vi "Panel Get Dryer Weight.vi"(0 "VISA resource name":refnum<visa-resource-name>, 2 "Agilent Scale?":bool, 11 "error in (no error)":errorcluster) -> (4 "VISA resource name out":refnum<visa-resource-name>, 6 "Empty Dryer Cold Weight":dbl, 8 "Init Scale Temp":dbl, 15 "error out":errorcluster)   [LabVIEW 2009]
uses:
  Global Test Variables DPT.vi
panel:
  out "Error Message":string
  in  "stop":bool
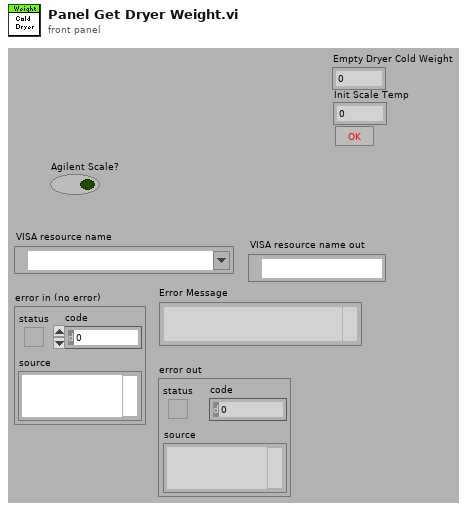
[diagram p1: front panel]
types:
  T1 = typedef "DPT Global Type.ctl" = cluster{"Test Setup":cluster{"RH Resistor":dbl, "Temp Cal":dbl, "Temp Coeff":dbl, "Power On Threshold":dbl, "MA Filter Size":i32, "Weight Offset":dbl, "Temp Resistor":dbl, "Gas Enabled":bool, "Gas P. Resistor":dbl, "Scale Com":dbl, "W. Samps":i32, "Temp4mA Val":dbl, "Temp20mA Val":dbl, "RH4mA Val":dbl, "RH20mA Val":dbl, "GPres4mA Val":dbl, "Gpres20mA Val":dbl}, "Agilent Setup":cluster{"Scale Channel":string, "TC Channels":string, "VDC Discrete Channels":string, "RH Chan":string, "Temp Chan":string, "Tscale Channel":string, "RDB Channel":string, "Gas Temperature":string, "Gas Pressure":string, "Barometric Pressure":string, "Gas Feedback Chan":string}, "Directories":cluster{"Work File Directory":path, "Save File Directory":path, "Library Directory":path, "Data Backup Directory":path, "Data Backup Dir Fail":path, "Lab Directory":path}, "Test Information":cluster{"Model:":string, "Temperature:":string, "Engineer:":string, "Technician:":string, "Comments:":string, "Lab ID:":string, "TR Number:":string, "Test Number:":string, "Test Station:":string, "Empty Dryer Cold Weight:":dbl, "Serial Number:":string, "Build:":string, "Dryer Type":string, "Humidity":string, "Test Title per TR:":string}, "cDAQ Array Locations":cluster{"Scale Channel":string, "TC Channels":string, "VDC Discrete Channel":string, "RH Chan":string, "Temp Chan":string, "Tscale Channel":string, "RDB Channel":string, "Gas Temperature":string, "Gas Pressure":string, "Barometric Pressure":string, "Gas Feedback Chan":string}}
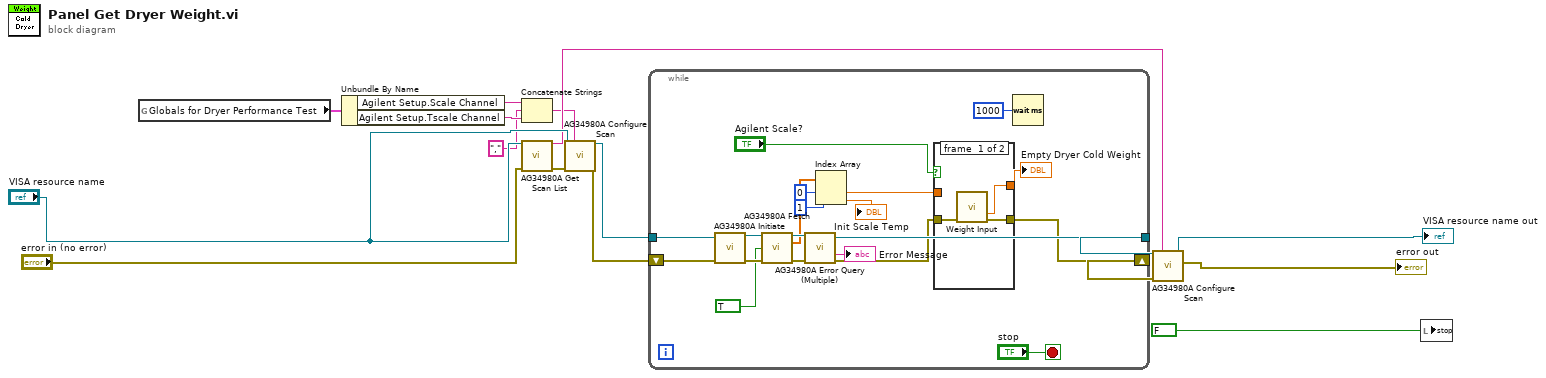
[diagram p0: block diagram]
diagram:
  n1 = global read "Global Test Variables DPT.vi" "Globals for Dryer Performance Test"() -> (w5:T1)
  n2 = Unbundle By Name(w5) -> ("Agilent Setup.Scale Channel"=w4:string, "Agilent Setup.Tscale Channel"=w3:string)
  n3 = Concatenate Strings(w4, "," ("string"), w3) -> (w1:string)
  n4 = call "AG34980A Get Scan List.vi"("VISA resource name"="VISA resource name", "error in (no error)"="error in (no error)") -> ("Channel List"=w6:string, "error out"=w10:errorcluster)  [unwired: 11 in, 1 out]
  n5 = call "AG34980A Configure Scan.vi"("VISA resource name"="VISA resource name", "Scan List(empty)"=w1, "error in (no error)"=w10) -> ("VISA resource name out"=w9:refnum<visa-resource-name>, "error out"=w11:errorcluster)  [unwired: 11 in]
  n6 = while {
    shift-right: [w17] -> w8
    shift-left: w11 -> [w31]
    tunnel: w9 -> [w30]
    tunnel: [w29] -> w7
    stop <- "stop" stop-if-true
    n7 = call "AG34980A Initiate.vi"("VISA resource name"=w30, "error in (no error)"=w31) -> ("VISA resource name out"=w34:refnum<visa-resource-name>, "error out"=w36:errorcluster)  [unwired: 12 in]
    n8 = call "AG34980A Fetch.vi"("VISA resource name"=w34, "Numbers Only (T:On)"=TRUE, "error in (no error)"=w36) -> ("VISA resource name out"=w33:refnum<visa-resource-name>, "Output Data (Numbers Only)"=w28:dbl[], "error out"=w35:errorcluster)  [unwired: 8 in, 2 out]
    n9 = call "AG34980A Error Query (Multiple).vi"("VISA resource name"=w33, "error in (no error)"=w35) -> ("VISA resource name out"=w29:refnum<visa-resource-name>, "Error Message"=→"Error Message":string, "error out"=w18:errorcluster)  [unwired: 10 in, 1 out]
    n10 = Index Array(array=w28, index #1=0 ("index"), index #2=1 ("index")) -> (element #1=w19:dbl, element #2=→"Init Scale Temp":dbl)
    n11 = case shown="False" "Agilent Scale?" {
      tunnel: [w37 w41] -> w20
      tunnel: w19 -> [_ w41]
      tunnel: w18 -> [w39 w40]
      tunnel: [w38 w40] -> w17
      frame #0 {
        n12 = call "Weight Input.vi"("Error In"=w39) -> ("Ave in Median Range"=w37:dbl, "error out"=w38:errorcluster)  [unwired: 10 in, 3 out]
      }
      frame #1 {
      }
    }
    "Empty Dryer Cold Weight" <- w20
    n13 = Wait (ms)(milliseconds to wait=u32 1000) -> ()  [unwired: 1 out]
  }
  n14 = call "AG34980A Configure Scan.vi"("VISA resource name"=w7, "Scan List(empty)"=w6, "error in (no error)"=w8) -> ("VISA resource name out"=→"VISA resource name out":refnum<visa-resource-name>, "error out"=→"error out":errorcluster)  [unwired: 11 in]
  n15 = local write "stop"(FALSE ("stop")) -> ()
